vi "SubVI_PM #.vi"(4 "Parameters":T1={"Number of Matches Requested"=1, "Minimum Match Score"=800.0, "Angle Ranges"=[]}, 5 "Algorithm":i32(ring) items=["All", "Low Discrepancy Sampling", "Grayscale Value Pyramid", "Gradients Pyramid"], 6 "Mode":u16(ring) items=["Find Reference", "Update CoordSys"], 7 "Template Image":T3, 8 "Error in":errorcluster, 9 "CoordSys In":T4 {"Measurement System"."Axis Reference" items=["Direct", "Indirect"]; "Measurement System"."Angle (deg)" format="%.2f"; "Measurement System"."Origin"."Y" format="%.2f"; "Measurement System"."Origin"."X" format="%.2f"; "Reference System"."Axis Reference" items=["Direct", "Indirect"]; "Reference System"."Angle (deg)" format="%.2f"; "Reference System"."Origin"."Y" format="%.2f"; "Reference System"."Origin"."X" format="%.2f"}, 10 "ROI_尋樣本":T5 {"Contours"."Type" items=["No Selection", "Point", "Line", "Rectangle", "Oval", "Polygon", "Freehand Region", "Annulus", "Unused2", "Unused3", "Broken Line", "Freehand Line", "Rotated Rectangle"]}, 11 "Image In":T3) -> (0 "Error out":errorcluster, 1 "CoordSys Out":T4 {"Measurement System"."Axis Reference" items=["Direct", "Indirect"]; "Measurement System"."Angle (deg)" format="%.2f"; "Measurement System"."Origin"."Y" format="%.2f"; "Measurement System"."Origin"."X" format="%.2f"; "Reference System"."Axis Reference" items=["Direct", "Indirect"]; "Reference System"."Angle (deg)" format="%.2f"; "Reference System"."Origin"."Y" format="%.2f"; "Reference System"."Origin"."X" format="%.2f"}, 2 "Matches":T2(array[cluster]) {"Bounding Box"."y" format="%.2f"; "Bounding Box"."x" format="%.2f"; "Position"."y" format="%.2f"; "Position"."x" format="%.2f"; "Score" format="%.2f"; "Scale" format="%.2f"; "Angle" format="%.2f"}, 3 "Image Out":T3)   [LabVIEW 2013]
uses:
  <vilib>/vision/Image Controls.llb/IMAQ Image.ctl
  <vilib>/vision/NI_Vision_Development_Module.lvlib
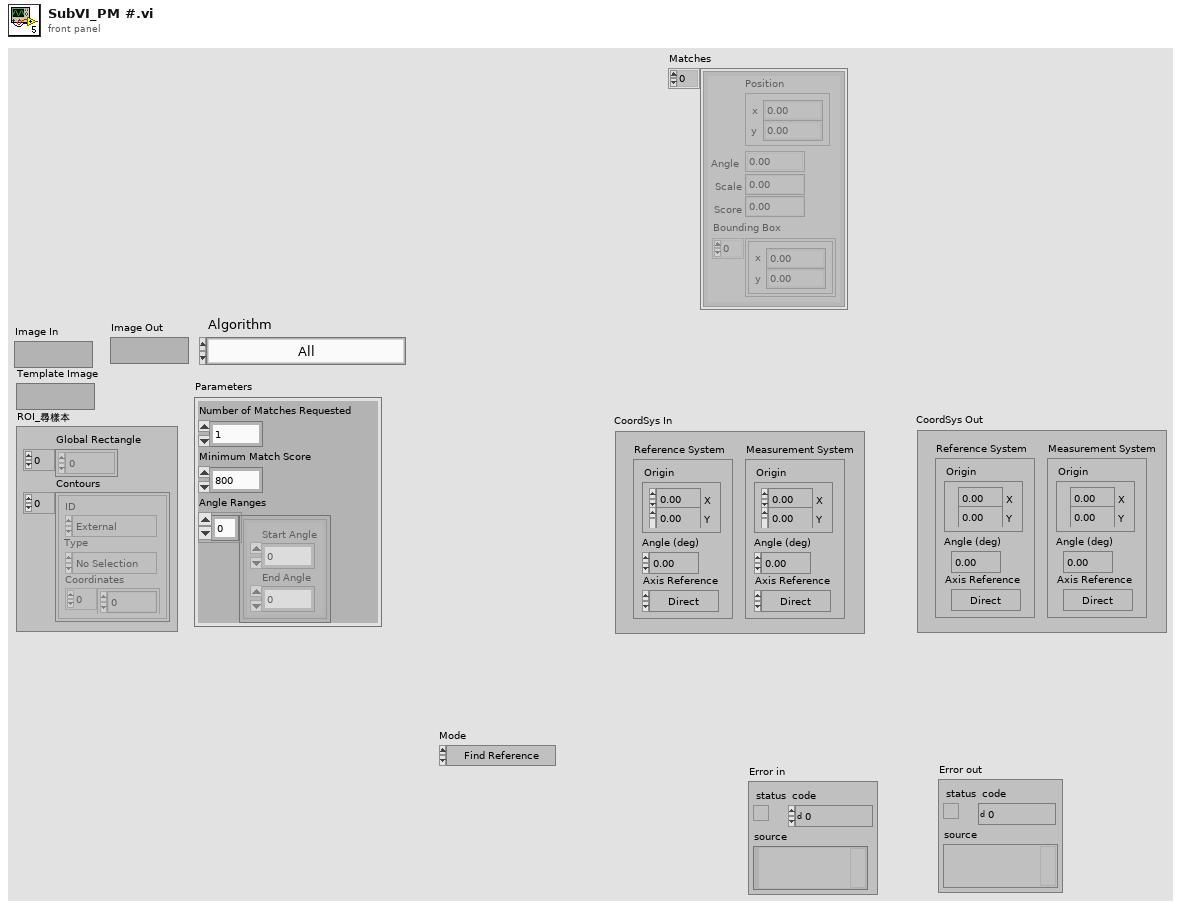
[diagram p1: front panel]
types:
  T1 = cluster{"Number of Matches Requested":i32, "Minimum Match Score":sgl, "Angle Ranges":cluster{"Start Angle":sgl, "End Angle":sgl}[]}
  T2 = cluster{"Position":cluster{"x":sgl, "y":sgl}, "Angle":sgl, "Scale":sgl, "Score":sgl, "Bounding Box":cluster{"x":sgl, "y":sgl}[]}[]
  T3 = typedef "IMAQ Image.ctl" = refnum<image>
  T4 = typedef "IMAQ Coordinate System" = cluster{"Reference System":cluster{"Origin":cluster{"X":sgl, "Y":sgl}, "Angle (deg)":sgl, "Axis Reference":u32}, "Measurement System":cluster{"Origin":cluster{"X":sgl, "Y":sgl}, "Angle (deg)":sgl, "Axis Reference":u32}}
  T5 = typedef "ROI Descriptor" = cluster{"Global Rectangle":i32[], "Contours":cluster{"ID":enum32{"External", "Internal"}, "Type":u32, "Coordinates":i32[]}[]}
  T6 = cluster{"Position":cluster{"x":sgl, "y":sgl}, "Angle":sgl, "Scale":sgl, "Score":sgl, "Bounding Box":cluster{"x":sgl, "y":sgl}[]}
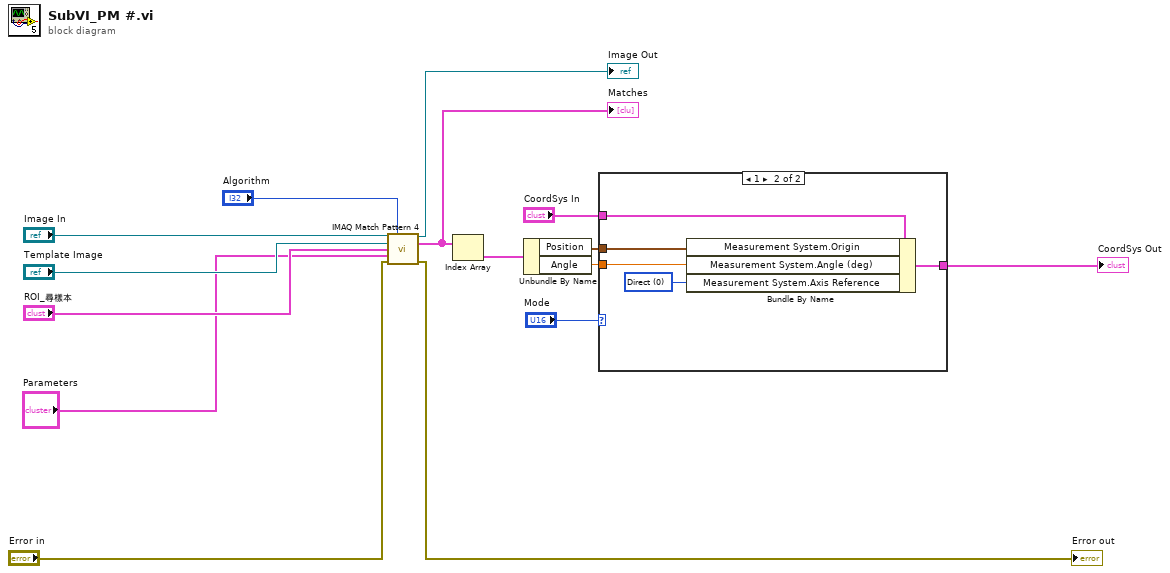
[diagram p0: block diagram]
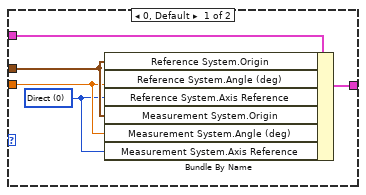
[diagram p2: hidden frame]
diagram:
  n1 = call "IMAQ Match Pattern 4"("Image"="Image In", "Algorithm"="Algorithm", "Template Image"="Template Image", "ROI Descriptor"="ROI_尋樣本", "Parameters"="Parameters", "error in (no error)"="Error in") -> ("Image (duplicate)"=→"Image Out":T3, "Matches (pixel)"=w3:T2, "error out"=→"Error out":errorcluster)  [unwired: 5 in, 2 out]
  "Matches" <- w3
  n2 = Index Array(array=w3) -> (element=w5:T6)  [unwired: 1 in]
  n3 = Unbundle By Name(w5) -> ("Position"=w11:cluster{"x":sgl, "y":sgl}, "Angle"=w10:sgl)
  n4 = case shown="1" "Mode" {
    tunnel: w11 -> [w18 w23]
    tunnel: [w20 w25] -> w6
    tunnel: w10 -> [w17 w22]
    tunnel: "CoordSys In" -> [w19 w24]
    frame 0, Default {
      w16 = u32 0 items=["Direct", "Indirect"] ("Axis Reference")
      n5 = Bundle By Name(cluster=w19, "Reference System.Origin"=w18, "Reference System.Angle (deg)"=w17, "Reference System.Axis Reference"=w16, "Measurement System.Origin"=w18, "Measurement System.Angle (deg)"=w17, "Measurement System.Axis Reference"=w16) -> (w20:T4)
    }
    frame 1 {
      w21 = u32 0 items=["Direct", "Indirect"] ("Axis Reference")
      n6 = Bundle By Name(cluster=w24, "Measurement System.Origin"=w23, "Measurement System.Angle (deg)"=w22, "Measurement System.Axis Reference"=w21) -> (w25:T4)
    }
  }
  "CoordSys Out" <- w6
